vi "Acq-module-5752.vi"(5 "IntermediateFIFO":refnum<k21>="FIFO0", 7 "AI Cluster":T1={"FPGA_AI3"="IO Module\\AI 1 Data N", "FPGA_AI2"="IO Module\\AI 1 Data N", "FPGA_AI1"="IO Module\\AI 1 Data N", "FPGA_AI0"="IO Module\\AI 1 Data N", "FPGA_AI7"="IO Module\\AI 1 Data N", "FPGA_AI6"="IO Module\\AI 1 Data N", "FPGA_AI5"="IO Module\\AI 1 Data N", "FPGA_AI4"="IO Module\\AI 1 Data N", "FPGA_AI11"="IO Module\\AI 1 Data N", "FPGA_AI10"="IO Module\\AI 1 Data N", "FPGA_AI9"="IO Module\\AI 1 Data N", "FPGA_AI8"="IO Module\\AI 1 Data N"}, 8 "NumChannels":T2, 9 "SamplingRate0":u16, 11 "Cluster in":T4={0, 0, 0, 0, 0, 0, 0, TRUE, TRUE, 0, 0, 0}) -> (1 "Analog Out Cluster":T3, 3 "cluster out":T4)   [LabVIEW 2013]
uses:
  N Channels 5752.ctl
  <vilib>/rvi/DataTransferAndStorage/Container/Common/niFpgaContainerExecOnDevCompGetState.vi
  <vilib>/rvi/FIFO/Fifo_Resource/nirvififoEmulationWriteFpgaImpl.vi
  <vilib>/rvi/DataTransferAndStorage/Container/Common/niFpgaContainerGetUniqueNameForEmu.vi
  <vilib>/rvi/interface/RandomDataEmulation/nirviRandomDataFPGAFIFO.vi
  <vilib>/rvi/interface/RandomDataEmulation/niFpgaRandomDataHandleErrors.vi
  <vilib>/rvi/eio/common/nirviEmuReportErrorAndStop.vi
  <vilib>/rvi/eio/common/nirviEmuTemplateMethod_errors.vi
  <vilib>/rvi/DataTransferAndStorage/Container/XNode/niFpgaContainer.xnode
  <vilib>/rvi/FIFO/Fifo_Resource/niFpgaFifoEmulationRefIn.vi
  <vilib>/eio/EIONode/EIONode.xnode
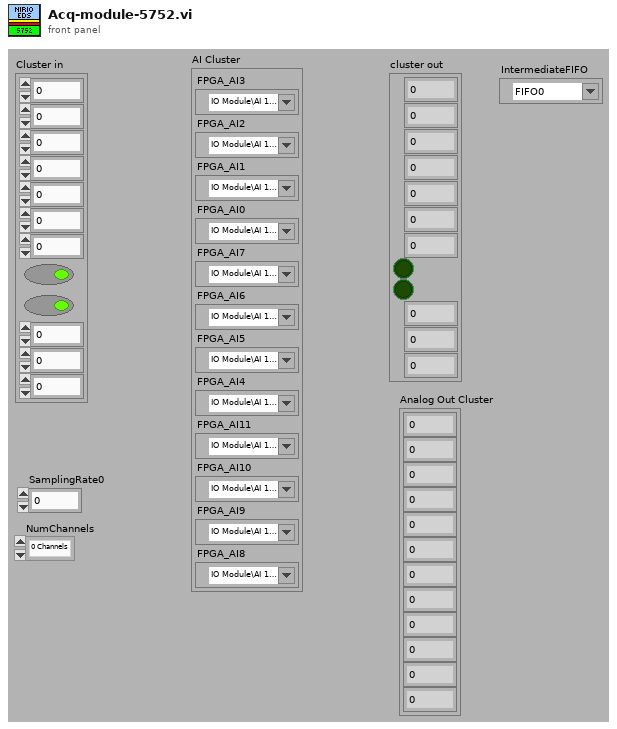
[diagram p1: front panel]
types:
  T1 = cluster{"FPGA_AI3":refnum<k21>, "FPGA_AI2":refnum<k21>, "FPGA_AI1":refnum<k21>, "FPGA_AI0":refnum<k21>, "FPGA_AI7":refnum<k21>, "FPGA_AI6":refnum<k21>, "FPGA_AI5":refnum<k21>, "FPGA_AI4":refnum<k21>, "FPGA_AI11":refnum<k21>, "FPGA_AI10":refnum<k21>, "FPGA_AI9":refnum<k21>, "FPGA_AI8":refnum<k21>}
  T2 = typedef "N Channels 5752.ctl" = enum16{"0 Channels", "1 Channels", "2 Channels", "3 Channels", "4 Channels", "5 Channels", "6 Channels", "7 Channels", "8 Channels", "9 Channels", "10 Channels", "11 Channels", "12 Channels"}
  T3 = cluster{i16, i16, i16, i16, i16, i16, i16, i16, i16, i16, i16, i16}
  T4 = cluster{u16, u16, u64, u64, u64, u64, i16, bool, bool, u64, u16, u16}
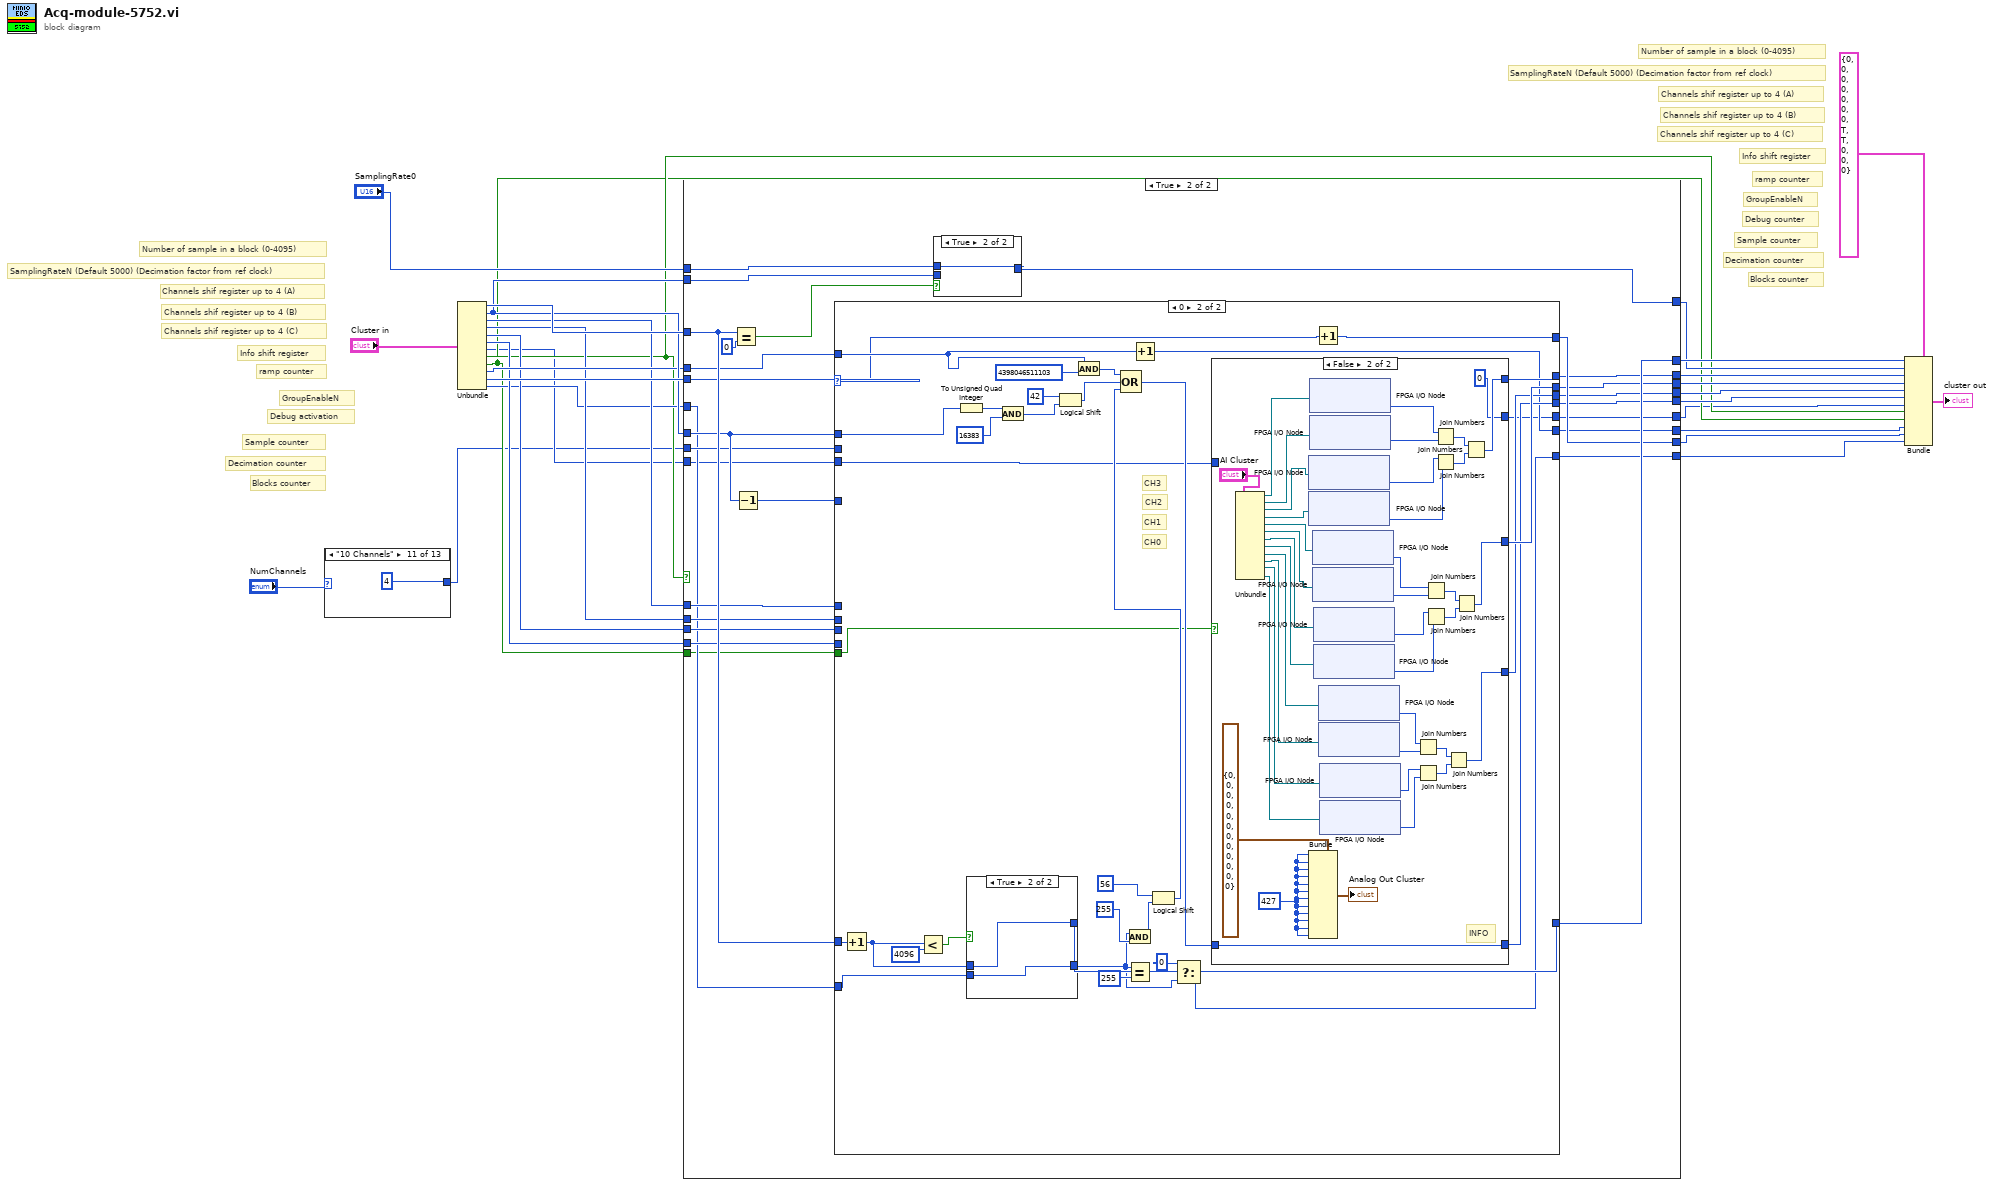
[diagram p0: block diagram]
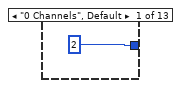
[diagram p2: hidden frame]
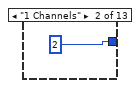
[diagram p3: hidden frame]
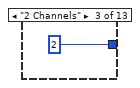
[diagram p4: hidden frame]
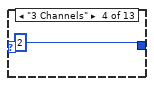
[diagram p5: hidden frame]
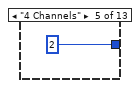
[diagram p6: hidden frame]
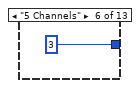
[diagram p7: hidden frame]
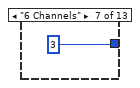
[diagram p8: hidden frame]
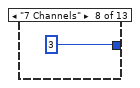
[diagram p9: hidden frame]
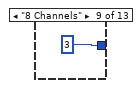
[diagram p10: hidden frame]
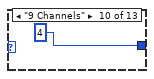
[diagram p11: hidden frame]
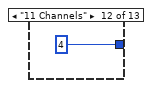
[diagram p12: hidden frame]
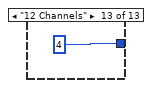
[diagram p13: hidden frame]
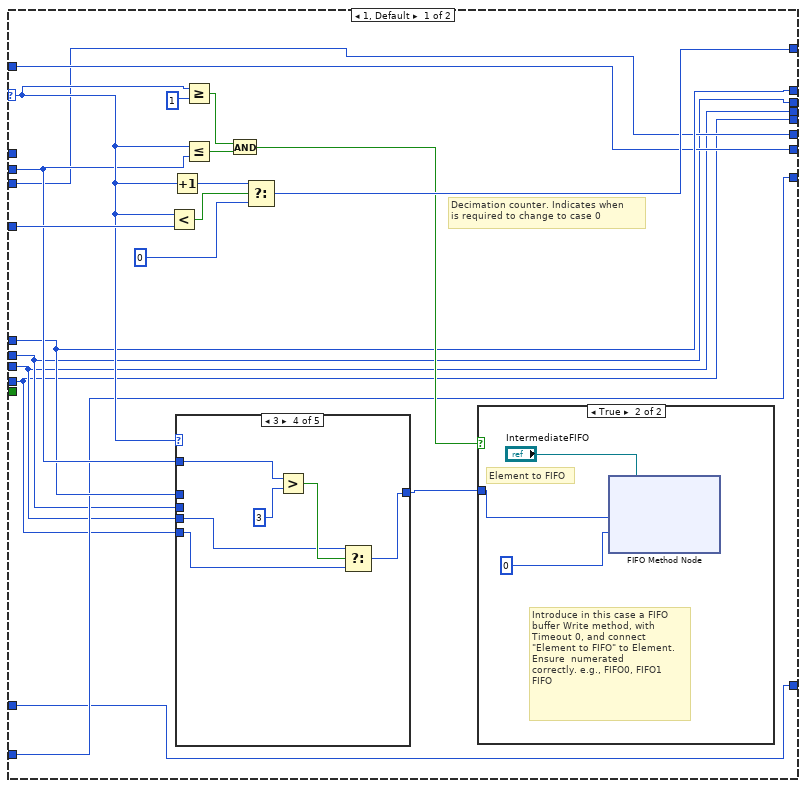
[diagram p15: hidden frame]
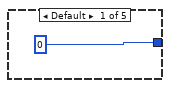
[diagram p17: hidden frame]
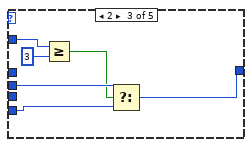
[diagram p19: hidden frame]
diagram:
  # "Blocks counter"
  # "Decimation counter"
  # "Blocks counter"
  # "Sample counter"
  # "Debug counter"
  # "ramp counter"
  # "Info shift register"
  # "Channels shif register up to 4 (C)"
  # "Channels shif register up to 4 (B)"
  # "Channels shif register up to 4 (A)"
  # "SamplingRateN (Default 5000) (Decimation factor from ref clock)"
  # "Number of sample in a block (0-4095)"
  # "GroupEnableN"
  # "Decimation counter"
  # "Sample counter"
  # "Debug activation"
  # "ramp counter"
  # "Info shift register"
  # "Channels shif register up to 4 (C)"
  # "Channels shif register up to 4 (B)"
  # "Channels shif register up to 4 (A)"
  # "SamplingRateN (Default 5000) (Decimation factor from ref clock)"
  # "Number of sample in a block (0-4095)"
  # "GroupEnableN"
  n1 = case shown="\"10 Channels\"" "NumChannels" {
    tunnel: [u8 2 ("Number of words") u8 2 ("Number of words") u8 2 ("Number of words") u8 2 ("Number of words") u8 2 ("Number of words") u8 3 ("Number of words") u8 3 ("Number of words") u8 3 ("Number of words") u8 3 ("Number of words") u8 4 ("Number of words") u8 4 ("Number of words") u8 4 ("Number of words") u8 4 ("Number of words")] -> w2
    frame "0 Channels", Default {
    }
    frame "1 Channels" {
    }
    frame "2 Channels" {
    }
    frame "3 Channels" {
    }
    frame "4 Channels" {
    }
    frame "5 Channels" {
    }
    frame "6 Channels" {
    }
    frame "7 Channels" {
    }
    frame "8 Channels" {
    }
    frame "9 Channels" {
    }
    frame "10 Channels" {
    }
    frame "11 Channels" {
    }
    frame "12 Channels" {
    }
  }
  n2 = Unbundle("Cluster in") -> (w28:u16, w15:u16, w12:u64, w11:u64, w10:u64, w9:u64, w4:i16, w6:bool, w5:bool, w14:u64, w21:u16, w8:u16)
  n3 = case shown="True" w6 {
    tunnel: w28 -> [w49 w74]
    tunnel: "SamplingRate0" -> [_ w77]
    tunnel: w15 -> [w50 w75]
    tunnel: [w49 w73] -> w25
    tunnel: [w50 w72] -> w24
    tunnel: w15 -> [_ w71]
    tunnel: w2 -> [_ w69]
    tunnel: w21 -> [w51 w68]
    tunnel: [w51 w67] -> w20
    tunnel: [w48 w66] -> w19
    tunnel: [w47 w65] -> w18
    tunnel: [w46 w64] -> w17
    tunnel: [w45 w63] -> w16
    tunnel: w14 -> [w44 w62]
    tunnel: [w44 w61] -> w13
    tunnel: w12 -> [w48 w60]
    tunnel: w11 -> [w47 w59]
    tunnel: w10 -> [w46 w58]
    tunnel: w9 -> [w45 w57]
    tunnel: w8 -> [w43 w56]
    tunnel: [w43 w55] -> w7
    tunnel: w5 -> [_ w54]
    tunnel: w4 -> [w42 w53]
    tunnel: [w42 w52] -> w3
    frame False {
    }
    frame True {
      n4 = Equal?(x=w74, y=u16 0) -> (x = y?=w76:bool)
      n5 = Decrement(x=w71) -> (x-1=w70:u16)
      n6 = case shown="0" w68 {
        selector: w68 -> [w90 w118]
        tunnel: w74 -> [w83 w151]
        tunnel: [w83 w147] -> w73
        tunnel: w71 -> [_ w144]
        tunnel: w70 -> [w93 _]
        tunnel: w69 -> [w89 _]
        tunnel: [w92 w117] -> w67
        tunnel: [w87 w131] -> w66
        tunnel: [w81 w130] -> w65
        tunnel: [w80 w129] -> w64
        tunnel: [w79 w128] -> w63
        tunnel: w62 -> [w85 w126]
        tunnel: [w85 w125] -> w61
        tunnel: w60 -> [w87 _]
        tunnel: w59 -> [w81 _]
        tunnel: w58 -> [w80 _]
        tunnel: w57 -> [w79 _]
        tunnel: w56 -> [w84 w124]
        tunnel: [w84 w123] -> w55
        tunnel: w54 -> [_ w122]
        tunnel: w53 -> [w82 w121]
        tunnel: [w82 w120] -> w52
        frame 1, Default {
          # "Decimation counter. Indicates when \nis required to change to case 0"
          n7 = Less?(x=w90, y=w93) -> (x < y?=w86:bool)
          n8 = Increment(x=w90) -> (x+1=w98:u16)
          n9 = case shown="3" w90 {
            tunnel: [u64 0 ("Element") w103 w106 w110 w116] -> w91
            tunnel: w87 -> [_ w103 _ _ _]
            tunnel: w81 -> [_ _ w109 _ _]
            tunnel: w80 -> [_ _ _ w112 _]
            tunnel: w79 -> [_ _ w105 w111 w116]
            tunnel: w89 -> [_ _ w108 w115 _]
            frame Default {
            }
            frame 1 {
            }
            frame 2 {
              n10 = Greater Or Equal?(x=w108, y=u8 3) -> (x >= y?=w104:bool)
              n11 = Select(t=w109, s=w104, f=w105) -> (s? t:f=w106:u64)
            }
            frame 3 {
              n12 = Greater?(x=w115, y=u8 3) -> (0:w113:bool)
              n13 = Select(t=w112, s=w113, f=w111) -> (s? t:f=w110:u64)
            }
            frame 4 {
            }
          }
          n14 = Greater Or Equal?(x=w90, y=u16 1) -> (x >= y?=w95:bool)
          n15 = Less Or Equal?(x=w90, y=w89) -> (x <= y?=w94:bool)
          n16 = And(x=w95, y=w94) -> (x .and. y?=w88:bool)
          n17 = Select(t=w98, s=w86, f=u16 0) -> (s? t:f=w92:u16)
          n18 = case shown="True" w88 {
            tunnel: w91 -> [_ w101]
            frame False {
            }
            frame True {
              # "Element to FIFO"
              # "Introduce in this case a FIFO buffer Write method, with Timeout 0, and connect \"Element to FIFO\" to Element. Ensure  numerated\ncorrectly. e.g., FIFO0, FIFO1 \nFIFO"
              n19 = xnode ("FIFO Method Node")("Element"=w101, "Timeout"=0, "FIFO In"="IntermediateFIFO") -> ()  [unwired: 2 out]
            }
          }
        }
        frame 0 {
          # "CH0"
          # "CH1"
          # "CH2"
          # "CH3"
          n20 = Increment(x=w151) -> (x+1=w148:u16)
          n21 = Less?(x=w148, y=u16 4096) -> (x < y?=w149:bool)
          n22 = To Unsigned Quad Integer(1:w144) -> (0:w146:u64)
          n23 = case shown="True" w149 {
            tunnel: w148 -> [_ w234]
            tunnel: [u16 0 w234] -> w147
            tunnel: w124 -> [w231 w233]
            tunnel: [w230 w233] -> w119
            frame False {
              n24 = Increment(x=w231) -> (x+1=w230:u16)
            }
            frame True {
            }
          }
          n25 = And(x=w146, y=i16 16383) -> (x .and. y?=w143:u64)
          n26 = Logical Shift(y=i8 42, x=w143) -> (x << y=w139:u64)
          n27 = And(x=w126, y=u64 4398046511103) -> (x .and. y?=w140:u64)
          n28 = And(x=w119, y=u64 255) -> (x .and. y?=w137:u64)
          n29 = Equal?(x=w119, y=u16 255) -> (x = y?=w134:bool)
          n30 = Increment(x=w126) -> (x+1=w125:u64)
          n31 = Logical Shift(y=i8 56, x=w137) -> (x << y=w132:u64)
          n32 = Compound Arithmetic op=OR(w140, w139, w132) -> (w127:u64)
          n33 = Select(t=u16 0, s=w134, f=w119) -> (s? t:f=w123:u16)
          n34 = case shown="False" w122 {
            tunnel: [w155 w229] -> w131
            tunnel: [w154 w204] -> w130
            tunnel: [w153 w203] -> w129
            tunnel: [w152 w228] -> w128
            tunnel: w127 -> [w152 w228]
            tunnel: w121 -> [w157 _]
            tunnel: [w156 i16 0] -> w120
            frame True {
              n35 = Add(x=w157, y=i16 5) -> (x+y=w184:i16)
              n36 = Add(x=i16 10, y=w157) -> (x+y=w182:i16)
              n37 = Add(x=w157, y=i16 15) -> (x+y=w180:i16)
              n38 = Add(x=w157, y=i16 20) -> (x+y=w169:i16)
              n39 = Add(x=w157, y=i16 25) -> (x+y=w174:i16)
              n40 = Add(x=i16 30, y=w157) -> (x+y=w172:i16)
              n41 = Add(x=w157, y=i16 35) -> (x+y=w170:i16)
              n42 = Add(x=w157, y=i16 40) -> (x+y=w159:i16)
              n43 = Add(x=w157, y=i16 45) -> (x+y=w164:i16)
              n44 = Add(x=i16 50, y=w157) -> (x+y=w162:i16)
              n45 = Add(x=w157, y=i16 55) -> (x+y=w160:i16)
              n46 = Less?(x=w157, y=i16 4095) -> (x < y?=w178:bool)
              n47 = Join Numbers(hi=w157, lo=w184) -> ((hi.lo)=w187:u32)
              n48 = Join Numbers(hi=w182, lo=w180) -> ((hi.lo)=w186:u32)
              n49 = Join Numbers(hi=w169, lo=w174) -> ((hi.lo)=w177:u32)
              n50 = Join Numbers(hi=w172, lo=w170) -> ((hi.lo)=w176:u32)
              n51 = Join Numbers(hi=w159, lo=w164) -> ((hi.lo)=w167:u32)
              n52 = Join Numbers(hi=w162, lo=w160) -> ((hi.lo)=w166:u32)
              n53 = Join Numbers(hi=w187, lo=w186) -> ((hi.lo)=w155:u64)
              n54 = Join Numbers(hi=w177, lo=w176) -> ((hi.lo)=w154:u64)
              n55 = Join Numbers(hi=w167, lo=w166) -> ((hi.lo)=w153:u64)
              n56 = case shown="True" w178 {
                tunnel: w157 -> [_ w190]
                tunnel: [i16 0 w189] -> w156
                frame False {
                }
                frame True {
                  n57 = Increment(x=w190) -> (x+1=w189:i16)
                }
              }
            }
            frame False {
              w225 = i16 427
              # "INFO"
              n58 = Unbundle("AI Cluster") -> ("FPGA_AI3"=w216:refnum<k21>, "FPGA_AI2"=w215:refnum<k21>, "FPGA_AI1"=w214:refnum<k21>, "FPGA_AI0"=w213:refnum<k21>, "FPGA_AI7"=w212:refnum<k21>, "FPGA_AI6"=w211:refnum<k21>, "FPGA_AI5"=w210:refnum<k21>, "FPGA_AI4"=w209:refnum<k21>, "FPGA_AI11"=w208:refnum<k21>, "FPGA_AI10"=w207:refnum<k21>, "FPGA_AI9"=w206:refnum<k21>, "FPGA_AI8"=w205:refnum<k21>)
              n59 = xnode "FPGA I/O Node"("FPGA I/O In"=w214) -> ("I/O Item"=w196:i16)  [unwired: 1 out]
              n60 = xnode "FPGA I/O Node"("FPGA I/O In"=w213) -> ("I/O Item"=w195:i16)  [unwired: 1 out]
              n61 = Bundle(cluster=T3 {0, 0, 0, 0, 0, 0, 0, 0, 0, 0, 0, 0} ("Cluster 2"), w225, w225, w225, w225, w225, w225, w225, w225, w225, w225, w225, w225) -> (→"Analog Out Cluster":T3)
              n62 = xnode "FPGA I/O Node"("FPGA I/O In"=w216) -> ("I/O Item"=w198:i16)  [unwired: 1 out]
              n63 = xnode "FPGA I/O Node"("FPGA I/O In"=w215) -> ("I/O Item"=w197:i16)  [unwired: 1 out]
              n64 = xnode "FPGA I/O Node"("FPGA I/O In"=w212) -> ("I/O Item"=w202:i16)  [unwired: 1 out]
              n65 = xnode "FPGA I/O Node"("FPGA I/O In"=w211) -> ("I/O Item"=w201:i16)  [unwired: 1 out]
              n66 = xnode "FPGA I/O Node"("FPGA I/O In"=w210) -> ("I/O Item"=w200:i16)  [unwired: 1 out]
              n67 = xnode "FPGA I/O Node"("FPGA I/O In"=w209) -> ("I/O Item"=w199:i16)  [unwired: 1 out]
              n68 = xnode "FPGA I/O Node"("FPGA I/O In"=w208) -> ("I/O Item"=w194:i16)  [unwired: 1 out]
              n69 = xnode "FPGA I/O Node"("FPGA I/O In"=w207) -> ("I/O Item"=w193:i16)  [unwired: 1 out]
              n70 = xnode "FPGA I/O Node"("FPGA I/O In"=w206) -> ("I/O Item"=w192:i16)  [unwired: 1 out]
              n71 = xnode "FPGA I/O Node"("FPGA I/O In"=w205) -> ("I/O Item"=w191:i16)  [unwired: 1 out]
              n72 = Join Numbers(hi=w194, lo=w193) -> ((hi.lo)=w218:u32)
              n73 = Join Numbers(hi=w192, lo=w191) -> ((hi.lo)=w219:u32)
              n74 = Join Numbers(hi=w202, lo=w201) -> ((hi.lo)=w220:u32)
              n75 = Join Numbers(hi=w200, lo=w199) -> ((hi.lo)=w221:u32)
              n76 = Join Numbers(hi=w198, lo=w197) -> ((hi.lo)=w222:u32)
              n77 = Join Numbers(hi=w196, lo=w195) -> ((hi.lo)=w223:u32)
              n78 = Join Numbers(hi=w218, lo=w219) -> ((hi.lo)=w203:u64)
              n79 = Join Numbers(hi=w220, lo=w221) -> ((hi.lo)=w204:u64)
              n80 = Join Numbers(hi=w222, lo=w223) -> ((hi.lo)=w229:u64)
            }
          }
          n81 = Increment(x=w118) -> (x+1=w117:u16)
        }
      }
      n82 = case shown="True" w76 {
        tunnel: w77 -> [_ w236]
        tunnel: [w235 w236] -> w72
        tunnel: w75 -> [w235 _]
        frame False {
        }
        frame True {
        }
      }
    }
  }
  n83 = Bundle(cluster=T4 {0, 0, 0, 0, 0, 0, 0, TRUE, TRUE, 0, 0, 0} ("Cluster in"), w25, w24, w19, w18, w17, w16, w3, w6, w5, w13, w20, w7) -> (→"cluster out":T4)
